vi "test-json-schema.vi"() -> ()   [LabVIEW 2019, in "JSON-Schema.lvlib" / "TEST-JSON-Schema.lvlib"]
uses:
  TEST-JSON-Schema.lvlib
  typedefs/test_cluster--cluster.ctl
  typedefs/test_enum--enum.ctl
  typedefs/test_nested_cluster--cluster.ctl
  JSON-Schema/JSON-Schema.lvlib
  <vilib>/JDP Science/JSONtext/JSONtext.lvlib
panel:
  in  "test object":enum16{"enum", "cluster", "nested cluster"}(ring)
  out "JSON Schema out":string
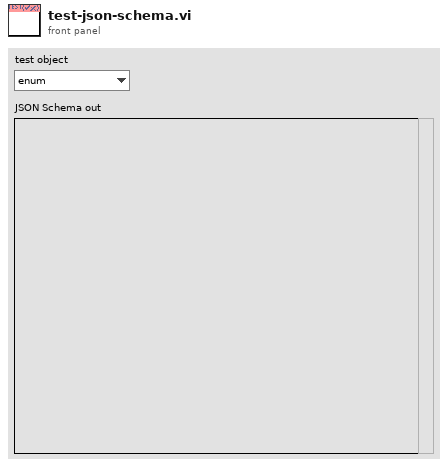
[diagram p1: front panel]
types:
  T1 = typedef "JSON-Schema.lvlib/TEST-JSON-Schema.lvlib/test_cluster--cluster.ctl" = cluster{"numeric":dbl, "test_enum":T2}
  T2 = typedef "JSON-Schema.lvlib/TEST-JSON-Schema.lvlib/test_enum--enum.ctl" = enum16{"option_1", "option_2"}
  T3 = typedef "JSON-Schema.lvlib/TEST-JSON-Schema.lvlib/test_nested_cluster--cluster.ctl" = cluster{"string":string, "test_cluster":T1}
  T4 = enum32{"Bad", "Idle", "Run top level", "Running"}
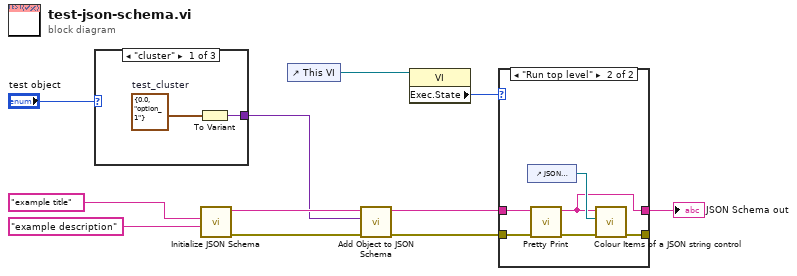
[diagram p0: block diagram]
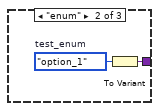
[diagram p2: hidden frame]
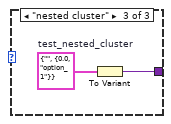
[diagram p3: hidden frame]
diagram:
  n1 = case shown="\"cluster\"" "test object" {
    tunnel: [w12 w14 w16] -> w4
    frame "cluster" {
      w13 = T1 {"numeric"=0.0, "test_enum"=enum."option_1"}  # test_cluster
      n2 = To Variant(anything=w13) -> (Variant=w12:variant)
    }
    frame "enum" {
      w15 = test_enum--enum."option_1"  # test_enum
      n3 = To Variant(anything=w15) -> (Variant=w14:variant)
    }
    frame "nested cluster" {
      w17 = T3 {"string"="", "test_cluster"={"numeric"=0.0, "test_enum"=enum."option_1"}}  # test_nested_cluster
      n4 = To Variant(anything=w17) -> (Variant=w16:variant)
    }
  }
  n5 = call "Initialize JSON Schema.vi"("Description"="example description", "Title"="example title") -> ("error out"=w5:errorcluster, "JSON Schema out"=w11:string)  [unwired: 8 in]
  n6 = control-ref of="This VI"() -> (w10:refnum<vi>)
  n7 = call "Add Object to JSON Schema.vi"("error in (no error)"=w5, "Object"=w4, "JSON Schema in"=w11) -> ("error out"=w6:errorcluster, "JSON Schema out"=w7:string)  [unwired: 7 in]
  n8 = property class="VI"(reference=w10) -> ("Exec.State"=w9:T4)  [unwired: 1 in, 2 out]
  n9 = case shown="\"Run top level\"" w9 {
    tunnel: w7 -> [w18 w25]
    tunnel: w6 -> [w19 w24]
    tunnel: [w19 w22] -> _
    tunnel: [w18 w20] -> w8
    frame Default {
    }
    frame "Run top level" {
      n10 = control-ref of="JSON Schema out"() -> (w21:refnum<vi>)
      n11 = call <vilib>:"Pretty Print.vi"("error in (no error)"=w24, "JSON"=w25) -> ("error out"=w23:errorcluster, "<JSON>"=w20:string)  [unwired: 7 in, 1 out]
      n12 = call <vilib>:"Colour Items of a JSON string control.vi"("error in (no error)"=w23, "String Control"=w21, "JSON"=w20) -> ("error out"=w22:errorcluster)  [unwired: 8 in]
    }
  }
  "JSON Schema out" <- w8
